vi "PmSensorSize.vi"(8 "error in (no error)":errorcluster, 11 "reference":refnum<k24>) -> (0 "error out":errorcluster, 1 "Height":u16, 2 "Width":u16, 3 "reference 2":refnum<k24>)   [LabVIEW 2022 SP3, in "Photometrics Camera.lvlib"]
uses:
  Photometrics Camera.lvlib
  C:/FlashGordon/Development/dll/PVCamNET.dll
  dll/PVCamNET.dll
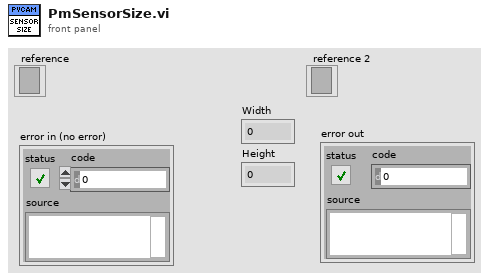
[diagram p1: front panel]
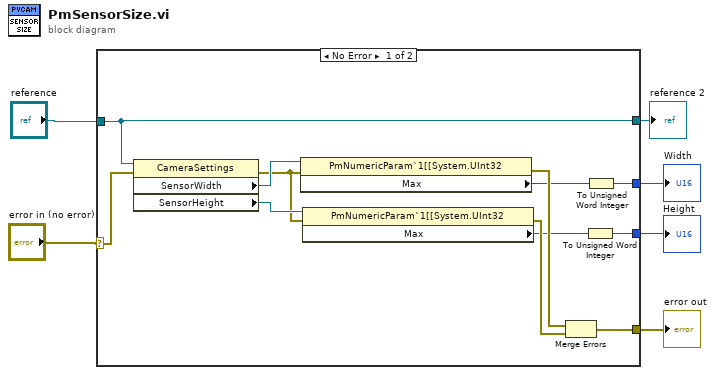
[diagram p0: block diagram]
diagram:
  n1 = case shown="No Error" "error in (no error)" {
    selector: "error in (no error)" -> [w12 w20]
    tunnel: [w10 _] -> w6
    tunnel: [w9 _] -> w5
    tunnel: [w11 w19] -> w1
    tunnel: [w13 w20] -> w4
    tunnel: "reference" -> [w11 w19]
    frame No Error {
      n2 = property class="CameraSettings"(reference=w11, error in=w12) -> (error out=w16:errorcluster, "SensorWidth"=w17:refnum<k24>, "SensorHeight"=w18:refnum<k24>)  [unwired: 1 out]
      n3 = property class="PmNumericParam`1[[System.UInt32"(reference=w17, error in=w16) -> (error out=w15:errorcluster, "Max"=w7:u32)  [unwired: 1 out]
      n4 = property class="PmNumericParam`1[[System.UInt32"(reference=w18, error in=w16) -> (error out=w14:errorcluster, "Max"=w8:u32)  [unwired: 1 out]
      n5 = Merge Errors(w15, w14) -> (w13:errorcluster)
      n6 = To Unsigned Word Integer(number=w8) -> (unsigned 16bit integer=w9:u16)
      n7 = To Unsigned Word Integer(number=w7) -> (unsigned 16bit integer=w10:u16)
    }
    frame Error {
    }
  }
  "Width" <- w6
  "Height" <- w5
  "error out" <- w4
  "reference 2" <- w1
